vi "_LV-TOML_Marshal.vi"   [LabVIEW 2020]
uses:
  <vilib>/LabVIEW Open Source Project/OpenSerializer/Serializer/Serializer.lvclass
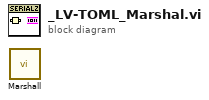
[diagram p0: block diagram]
diagram:
  n1 = call <vilib>:"Marshall.vi"() -> ()  [unwired: 9 in, 3 out]
